vi "Test Main.vi"(8 "Cluster In":T2, 9 "Numeric In":i32, 10 "Test In":T1, 11 "Test Class.lvclass In":refnum<class "Test Class.lvclass">) -> (0 "Cluster Out":T2, 2 "Test Out":T1, 3 "Test Class.lvclass Out":refnum<class "Test Class.lvclass">)   [LabVIEW 2020]
uses:
  Class/Test Class.lvclass
  Typdefs/Enum Test.ctl
  Typdefs/Cluster Test.ctl
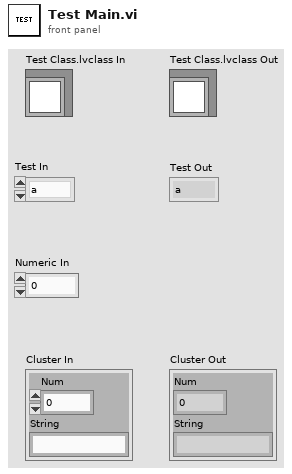
[diagram p1: front panel]
types:
  T1 = typedef "Enum Test.ctl" = enum16{"a", "b"}
  T2 = typedef "Cluster Test.ctl" = cluster{"Num":i32, "String":string}
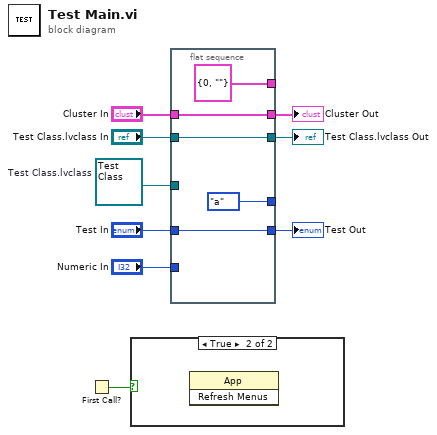
[diagram p0: block diagram]
diagram:
  w1 = refnum<class "Test Class.lvclass"> refnum  # Test Class.lvclass
  n1 = First Call?() -> (First Call?: T/F=w7:bool)
  n2 = case shown="True" w7 {
    frame False {
    }
    frame True {
      n3 = invoke class="App" method="Refresh Menus"() -> ()  [unwired: 3 in, 3 out]
    }
  }
  n4 = flat-sequence {
    tunnel: "Cluster In" -> [w14]
    tunnel: [w14] -> w8
    tunnel: "Numeric In" -> [_]
    tunnel: [Enum_Test."a"] -> _
    tunnel: [w11] -> w5
    tunnel: [w12] -> w2
    tunnel: "Test Class.lvclass In" -> [w12]
    tunnel: w1 -> [_]
    tunnel: "Test In" -> [w11]
    tunnel: [T2 {"Num"=0, "String"=""} ("Cluster")] -> _
    frame #0 {
    }
  }
  "Cluster Out" <- w8
  "Test Out" <- w5
  "Test Class.lvclass Out" <- w2
